vi "PLC.Dial800._TEST Set then Read Str Value.vi"() -> ()   [LabVIEW 2018]
panel:
  out "error out 2":errorcluster
  out "String 2":string
  in  "String":string
  in  "Write?":bool
  in  "data 2":i32
  out "Variant":variant
  out "timed out 2":bool
  out "timed out":bool
  in  "Boolean":bool
  out "timestamp":timestamp
  in  "wait for updated value (T)":bool
  in  "ms timeout (1000)":i32=1000
  out "quality":u64 format="%b"
  out "status":u32
  out "Value":bool
  out "error out":errorcluster
  in  "URL":string="opc://localhost/RSLinx OPC Server/[Stn800]Program:Stn001_90_OffloadMain.TestPC[0].Done"
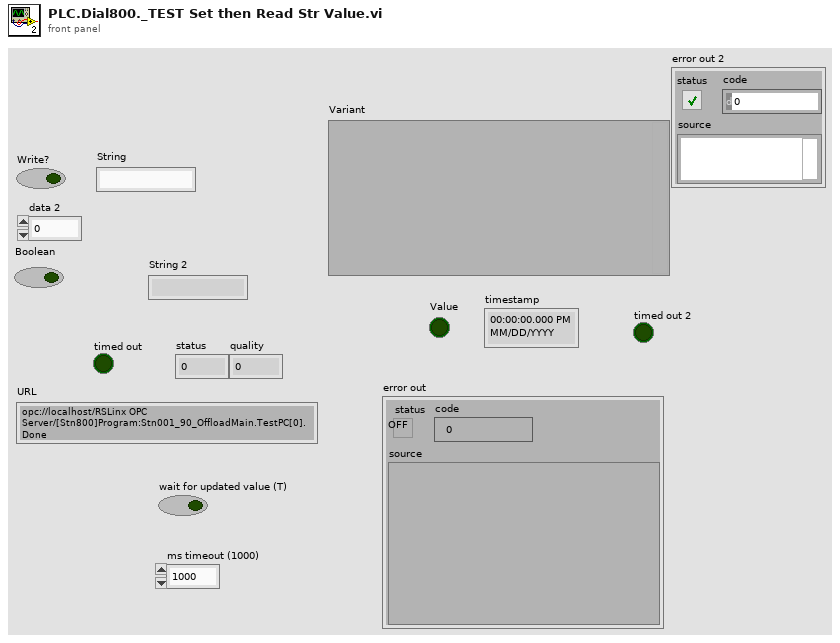
[diagram p1: front panel]
types:
  T1 = enum16{"Read", "Write", "ReadWrite", "BufferedRead", "BufferedReadWrite"}
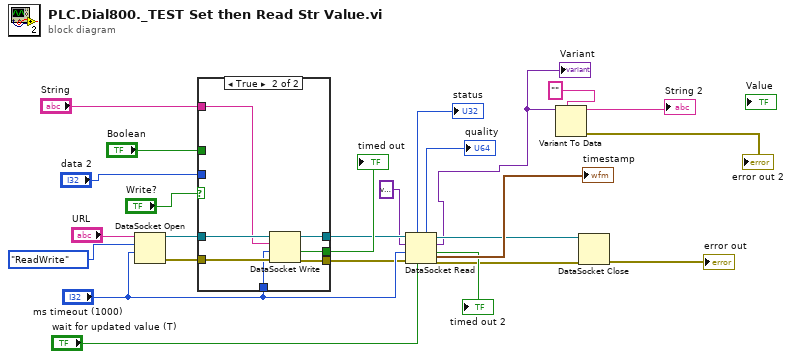
[diagram p0: block diagram]
diagram:
  n1 = DataSocket Open(9:"ms timeout (1000)", 10:T1."ReadWrite" ("mode"), 11:"URL") -> (0:w15:errorcluster, 3:w16:refnum<k13>)  [unwired: 1 in]
  n2 = case shown="True" "Write?" {
    tunnel: "Boolean" -> [_ _]
    tunnel: [_ w34] -> w20
    tunnel: [w27 w33] -> w18
    tunnel: w16 -> [w27 w32]
    tunnel: w15 -> [w26 w31]
    tunnel: "ms timeout (1000)" -> [_ w30]
    tunnel: [w26 w29] -> w9
    tunnel: "data 2" -> [_ _]
    tunnel: "String" -> [_ w28]
    frame False {
    }
    frame True {
      n3 = DataSocket Write(8:w31, 9:w30, 10:w28, 11:w32) -> (0:w29:errorcluster, 1:w34:bool, 3:w33:refnum<k13>)
    }
  }
  "timed out" <- w20
  n4 = DataSocket Read(6:"wait for updated value (T)", 8:w9, 9:"ms timeout (1000)", 10:variant, 11:w18) -> (0:w13:errorcluster, 1:→"timed out 2":bool, 2:w6:variant, 3:w14:refnum<k13>, 4:→"timestamp":timestamp, 5:→"quality":u64, 7:→"status":u32)
  "Variant" <- w6
  n5 = Variant To Data(type="", Variant=w6) -> (data=→"String 2":string, error out=→"error out 2":errorcluster)  [unwired: 1 in]
  n6 = DataSocket Close(8:w13, 11:w14) -> (0:→"error out":errorcluster)  [unwired: 1 in, 1 out]
